vi "Validate Fixed Header.vi"(8 "error in (no error)":errorcluster, 11 "SUBSCRIBE in":refnum<class "SUBSCRIBE.lvclass">) -> (0 "error out":errorcluster, 1 "Valid":bool, 3 "SUBSCRIBE out":refnum<class "SUBSCRIBE.lvclass">)   [LabVIEW 2013, in "SUBSCRIBE.lvclass"]
uses:
  SUBSCRIBE.lvclass
  ControlPacket/ControlPacket.lvclass/ControlPacket.ctl
  ControlPacket/ControlPacket.lvclass
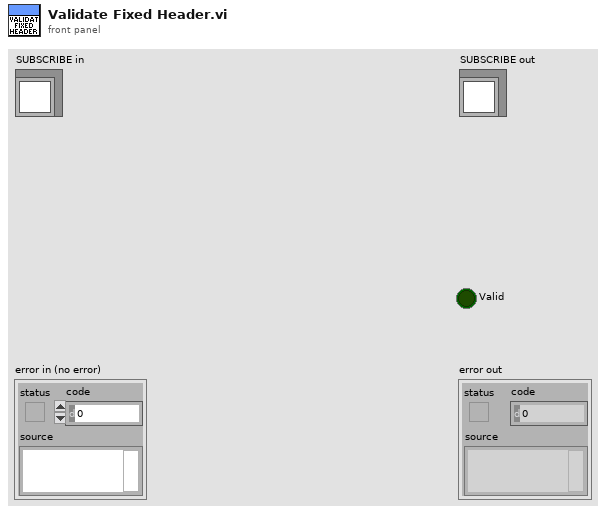
[diagram p1: front panel]
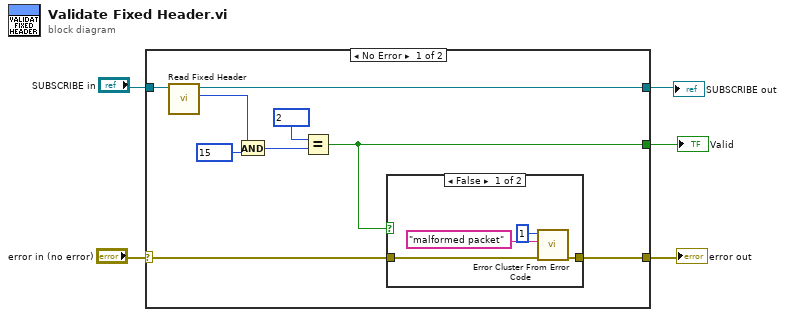
[diagram p0: block diagram]
diagram:
  n1 = case shown="No Error" "error in (no error)" {
    selector: "error in (no error)" -> [w7 w21]
    tunnel: [w6 w21] -> w3
    tunnel: [w8 _] -> w1
    tunnel: [w14 w20] -> w2
    tunnel: "SUBSCRIBE in" -> [w9 w20]
    frame No Error {
      n2 = call "Read Fixed Header.vi"("ControlPacket in"=w9) -> ("Fixed Header"=w12:u8, "ControlPacket out"=w14:refnum<class "SUBSCRIBE.lvclass">)  [unwired: 9 in]
      n3 = And(x=w12, y=u8 15) -> (x .and. y?=w11:u8)
      n4 = Equal?(x=u8 2 ("y"), y=w11) -> (x = y?=w8:bool)
      n5 = case shown="False" w8 {
        tunnel: [w16 w19] -> w6
        tunnel: w7 -> [w15 w19]
        frame False {
          n6 = call <vilib>:"Error Cluster From Error Code.vi"("error in (no error)"=w15, "error message (\"\")"="malformed packet" ("error message (\"\")"), "error code (0)"=1) -> ("error out"=w16:errorcluster)  [unwired: 6 in]
        }
        frame True {
        }
      }
    }
    frame Error {
    }
  }
  "Valid" <- w1
  "error out" <- w3
  "SUBSCRIBE out" <- w2
